vi "Calc CRC-sub.vi"(2 "Command":u16 format="%.0x", 3 "Adress":u16 format="%.0x", 4 "Data L":u16 format="%.0x", 5 "Data H":u16 format="%.0x", 6 "Reg L":u16 format="%.0x", 7 "Reg H":u16 format="%.0x") -> (0 "L byte":u8 format="%x", 1 "H byte":u8 format="%x")   [LabVIEW 2009]
panel:
  in  "Number of Byte":i32=6
  out "CRC":u16 format="%.0x"
  # "(HEX)"
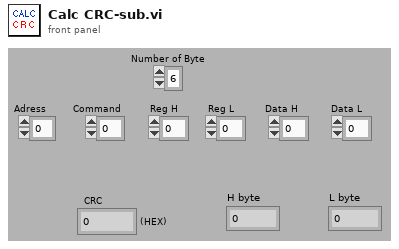
[diagram p1: front panel]
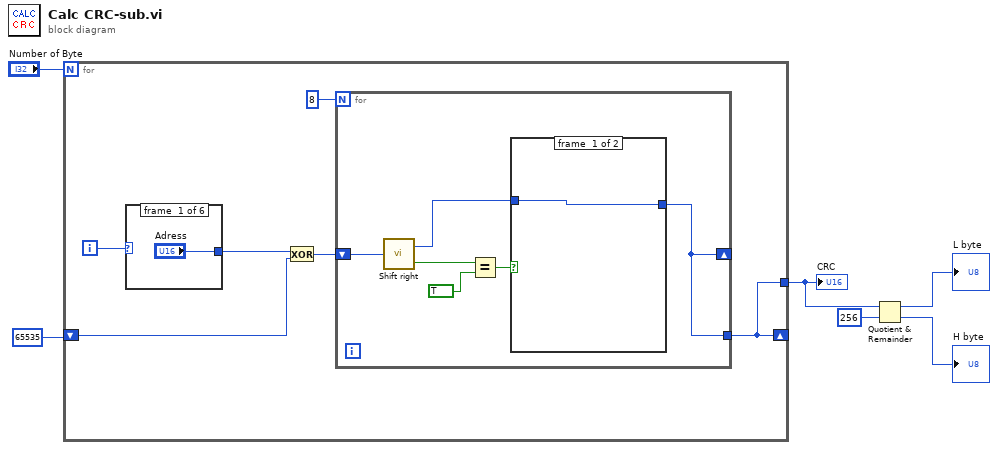
[diagram p0: block diagram]
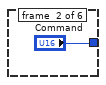
[diagram p2: hidden frame]
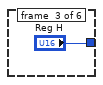
[diagram p3: hidden frame]
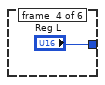
[diagram p4: hidden frame]
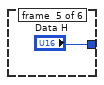
[diagram p5: hidden frame]
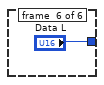
[diagram p6: hidden frame]
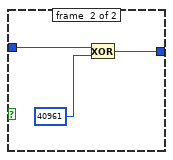
[diagram p7: hidden frame]
diagram:
  n1 = for {
    N: "Number of Byte" -> [_]
    shift-right: [w8] -> _
    shift-left: u16 65535 ("y") -> [w7]
    tunnel: [w8] -> w4
    i -> [w10]
    n2 = case shown="5" w10 {
      tunnel: ["Adress" "Command" "Reg H" "Reg L" "Data H" "Data L"] -> w9
      frame #0 {
      }
      frame #1 {
      }
      frame #2 {
      }
      frame #3 {
      }
      frame #4 {
      }
      frame #5 {
      }
    }
    n3 = Exclusive Or(1:w7, 2:w9) -> (0:w11:u16)
    n4 = for {
      N: 8 -> [_]
      shift-right: [w19] -> _
      shift-left: w11 -> [w22]
      tunnel: [w19] -> w8
      n5 = call "Shift right.vi"("Num In"=w22) -> ("Num Out"=w21:u16, "LSB"=w20:bool)
      n6 = Equal?(x=w20, y=TRUE) -> (x = y?=w23:bool)
      n7 = case shown="True" w23 {
        tunnel: w21 -> [w25 w27]
        tunnel: [w25 w26] -> w19
        frame #0 {
        }
        frame #1 {
          n8 = Exclusive Or(1:u16 40961 ("y"), 2:w27) -> (0:w26:u16)
        }
      }
    }
  }
  "CRC" <- w4
  n9 = Quotient & Remainder(x=w4, y=u16 256) -> (x-y*floor(x/y)=→"L byte":u16, floor(x/y)=→"H byte":u16)
